vi "single action.vi"() -> ()   [LabVIEW 2015]
uses:
  result/result.lvclass
  dispatcher/pool sizes.ctl
  result/result.lvclass/result.ctl
  result/get data.vi
  result/get error.vi
  result/get subresults.vi
  dispatcher/thread pool.lvclass
  standard reporters/event reporter/event reporter.lvclass
  standard action/wait action/wait action.lvclass
panel:
  out "x-y 2":dbl
  out "x-y":dbl
  out "subresults":refnum<class "result.lvclass">[](array[class])
  out "error":errorcluster
  out "data":variant
  out "Time":u32
  out "result":refnum<class "result.lvclass">
  out "error out":errorcluster
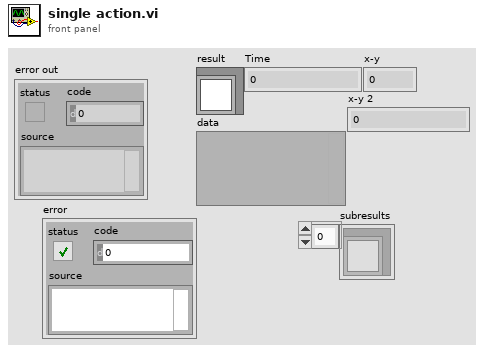
[diagram p1: front panel]
types:
  T1 = typedef "thread pool.lvclass/pool sizes.ctl" = cluster{"UI thread":u8, "standard":u8, "instrument I/O":u8, "data acquisition":u8, "other 1":u8, "other 2":u8}
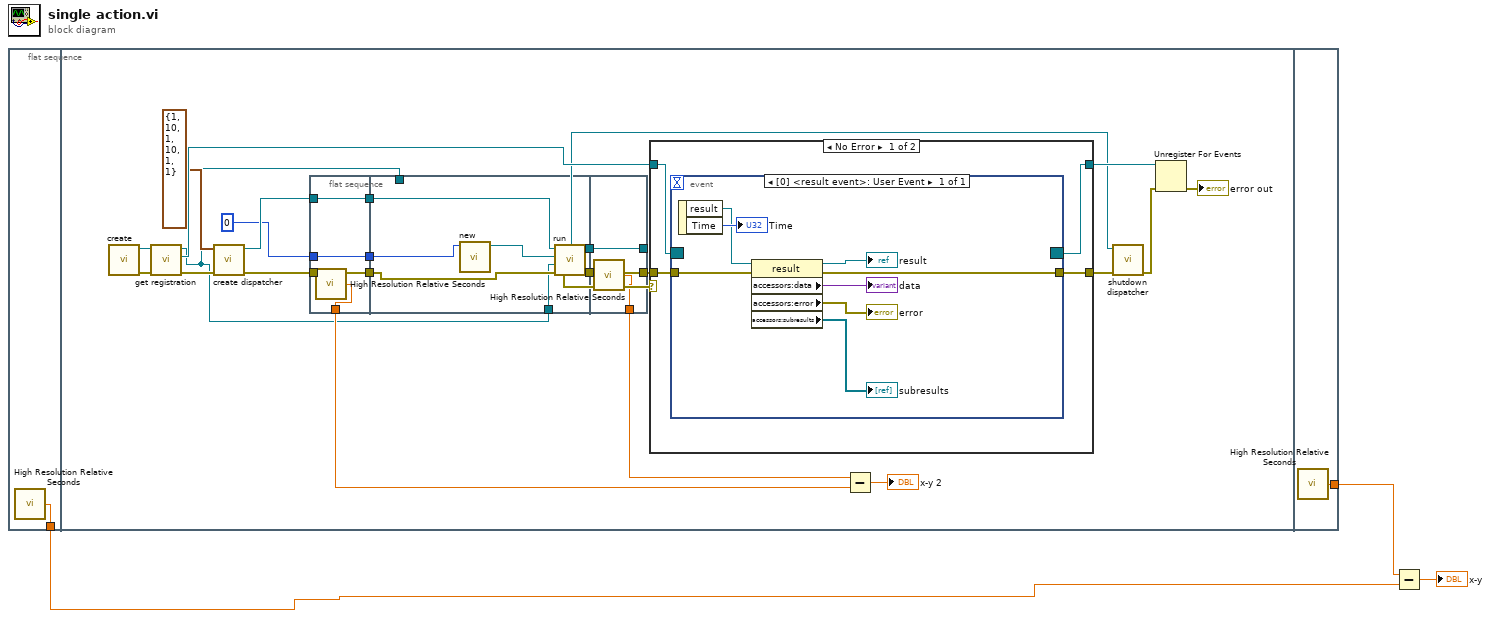
[diagram p0: block diagram]
diagram:
  n1 = flat-sequence {
    tunnel: [w4] -> w2
    tunnel: [w56] -> w3
    frame #0 {
      n2 = call <vilib>:"High Resolution Relative Seconds.vi"() -> ("relative seconds"=w4:dbl)
    }
    frame #1 {
      n3 = call "create.vi"() -> ("error out"=w23:errorcluster, "event reporter out"=w24:refnum<class "event reporter.lvclass">)  [unwired: 10 in]
      n4 = call "get registration.vi"("error in"=w23, "event reporter in"=w24) -> ("error out"=w22:errorcluster, "result registration"=w21:refnum<event-registration>, "event reporter out"=w5:refnum<class "event reporter.lvclass">)  [unwired: 7 in]
      n5 = call "create dispatcher.vi"("error in"=w22, "pool sizes (standard=10)"=T1 {"UI thread"=1, "standard"=10, "instrument I/O"=1, "data acquisition"=10, "other 1"=1, "other 2"=1} ("initial pool sizes")) -> ("error out"=w26:errorcluster, "dispatcher"=w27:refnum<class "thread pool.lvclass">)  [unwired: 8 in]
      n6 = flat-sequence {
        tunnel: 0 -> [w29]
        tunnel: w26 -> [w30]
        tunnel: w27 -> [w31]
        tunnel: [w31] -> w11
        tunnel: [w30] -> w10
        tunnel: [w29] -> w9
        tunnel: [w28] -> w7
        tunnel: [w37] -> w13
        tunnel: [w36] -> w12
        tunnel: w11 -> [w38]
        tunnel: w10 -> [w34]
        tunnel: w9 -> [w33]
        tunnel: w5 -> [_]
        tunnel: w5 -> [w32]
        tunnel: [w40] -> w15
        tunnel: [w41] -> w19
        tunnel: w13 -> [w41]
        tunnel: w12 -> [w40]
        tunnel: [w39] -> w8
        frame #0 {
          n7 = call <vilib>:"High Resolution Relative Seconds.vi"() -> ("relative seconds"=w28:dbl)
        }
        frame #1 {
          n8 = call "new.vi"("timer"=w33) -> ("wait action out"=w35:refnum<class "wait action.lvclass">)  [unwired: 10 in]
          n9 = call "run.vi"("error in"=w34, "results reporter"=w32, "task"=w35, "thread pool in"=w38) -> ("error out"=w36:errorcluster, "thread pool out"=w37:refnum<class "thread pool.lvclass">)  [unwired: 6 in]
        }
        frame #2 {
          n10 = call <vilib>:"High Resolution Relative Seconds.vi"() -> ("relative seconds"=w39:dbl)
        }
      }
      n11 = case shown="No Error" w15 {
        tunnel: w21 -> [w45 w55]
        tunnel: [w44 w55] -> w20
        tunnel: [w43 w54] -> w16
        tunnel: w15 -> [w42 w54]
        frame No Error {
          n12 = event shown="[0] <result event>: User Event" {
            selector: w45 -> [_]
            dyn-events: [_] -> w44
            timeout: _ -> [_]
            tunnel: [w51] -> w43
            tunnel: w42 -> [w52]
            event User Event {
              n13 = event-data() -> ("result"=w50:refnum<class "result.lvclass">, "Time"=→"Time":u32)  [unwired: 1 in]
              n14 = property class="result"(reference=w50, error in=w52) -> (reference out=→"result":refnum<class "result.lvclass">, error out=w51:errorcluster, "accessors:data"=→"data":variant, "accessors:error"=→"error":errorcluster, "accessors:subresults"=→"subresults":refnum<class "result.lvclass">[])
            }
          }
        }
        frame Error {
        }
      }
      n15 = Subtract(x=w8, y=w7) -> (x-y=→"x-y 2":dbl)
      n16 = call "shutdown dispatcher.vi"("error in"=w16, "thread pool"=w19) -> ("error out"=w18:errorcluster)  [unwired: 9 in]
      n17 = Unregister For Events(event registration refnum=w20, error in=w18) -> (error out=→"error out":errorcluster)
    }
    frame #2 {
      n18 = call <vilib>:"High Resolution Relative Seconds.vi"() -> ("relative seconds"=w56:dbl)
    }
  }
  n19 = Subtract(x=w3, y=w2) -> (x-y=→"x-y":dbl)
